vi "Create.vi"(8 "Error In":errorcluster, 11 "Process In":refnum<class "Process.lvclass">) -> (0 "Error Out":errorcluster, 3 "Process Out":refnum<class "Process.lvclass">)   [LabVIEW 2019, in "Process.lvclass"]
uses:
  Process.lvclass
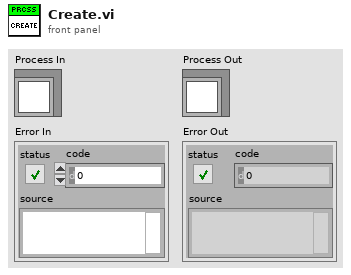
[diagram p1: front panel]
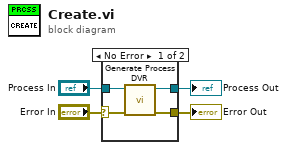
[diagram p0: block diagram]
diagram:
  n1 = case shown="No Error" "Error In" {
    selector: "Error In" -> [w7 w10]
    tunnel: [w5 w10] -> w3
    tunnel: "Process In" -> [w8 w9]
    tunnel: [w6 w9] -> w1
    frame No Error {
      n2 = call "Generate Process DVR.vi"("Error In"=w7, "Process In"=w8) -> ("Error Out"=w5:errorcluster, "Process Out"=w6:refnum<class "Process.lvclass">)  [unwired: 8 in]
    }
    frame Error {
    }
  }
  "Process Out" <- w1
  "Error Out" <- w3
